vi "Fast send and receive.vi"(10 "write to laser":string, 11 "VISA resource name":refnum<visa-resource-name>) -> (2 "read from laser":string, 3 "VISA resource name out":refnum<visa-resource-name>)   [LabVIEW 2017]
panel:
  # "This VI sends and receives commands to the laser.  This VI is used as the lower-level communication VI for the rest of the VIs included here."
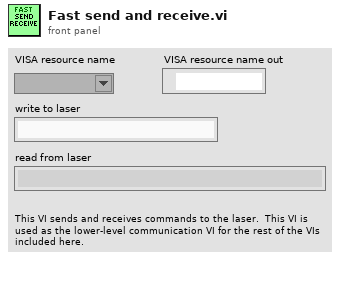
[diagram p1: front panel]
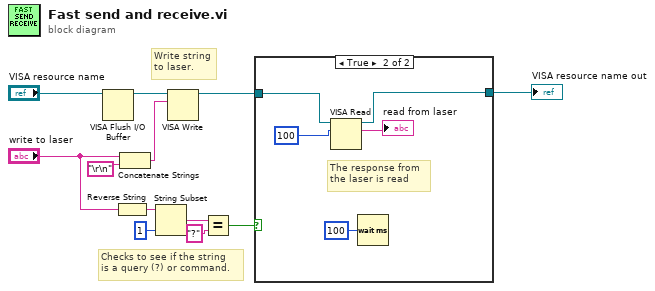
[diagram p0: block diagram]
diagram:
  # "Checks to see if the string\nis a query (?) or command."
  # "Write string\nto laser."
  n1 = VISA Flush I/O Buffer(VISA resource name="VISA resource name") -> (VISA resource name out=w4:refnum<visa-resource-name>)  [unwired: 2 in, 1 out]
  n2 = Reverse String(1:"write to laser") -> (0:w9:string)
  n3 = Concatenate Strings("write to laser", "\r\n") -> (w11:string)
  n4 = String Subset(string=w9, length (rest)=1 ("length (rest)")) -> (substring=w7:string)  [unwired: 1 in]
  n5 = VISA Write(VISA resource name=w4, write buffer=w11) -> (VISA resource name out=w10:refnum<visa-resource-name>)  [unwired: 1 in, 2 out]
  n6 = Equal?(x=w7, y="?") -> (x = y?=w5:bool)
  n7 = case shown="True" w5 {
    tunnel: w10 -> [w13 w16]
    tunnel: [w13 w14] -> w1
    frame False {
    }
    frame True {
      # "The response from\nthe laser is read"
      n8 = VISA Read(VISA resource name=w16, byte count=u32 100) -> (VISA resource name out=w14:refnum<visa-resource-name>, read buffer=→"read from laser":string)  [unwired: 1 in, 2 out]
      n9 = Wait (ms)(milliseconds to wait=u32 100) -> ()  [unwired: 1 out]
    }
  }
  "VISA resource name out" <- w1
